vi "TMjisuan.vi"() -> ()   [LabVIEW 2018]
uses:
  <vilib>/userdefined/High Color/IMAQdx.ctl
  <vilib>/vision/driver/NI_Vision_Acquisition_Software.lvlib
  <vilib>/vision/NI_Vision_Development_Module.lvlib
panel:
  out "Frame Rate":dbl
  out "Image Number":u32
  out "位置":string
  out "appended path":path
  out "Kobs":cdb[][](array[numeric])
  in  "Stop (F)":bool caption="亮度确认"
  in  "当前增益":u32=20000 caption="Gain::Value"
  out "输出":T1(plugin-control)
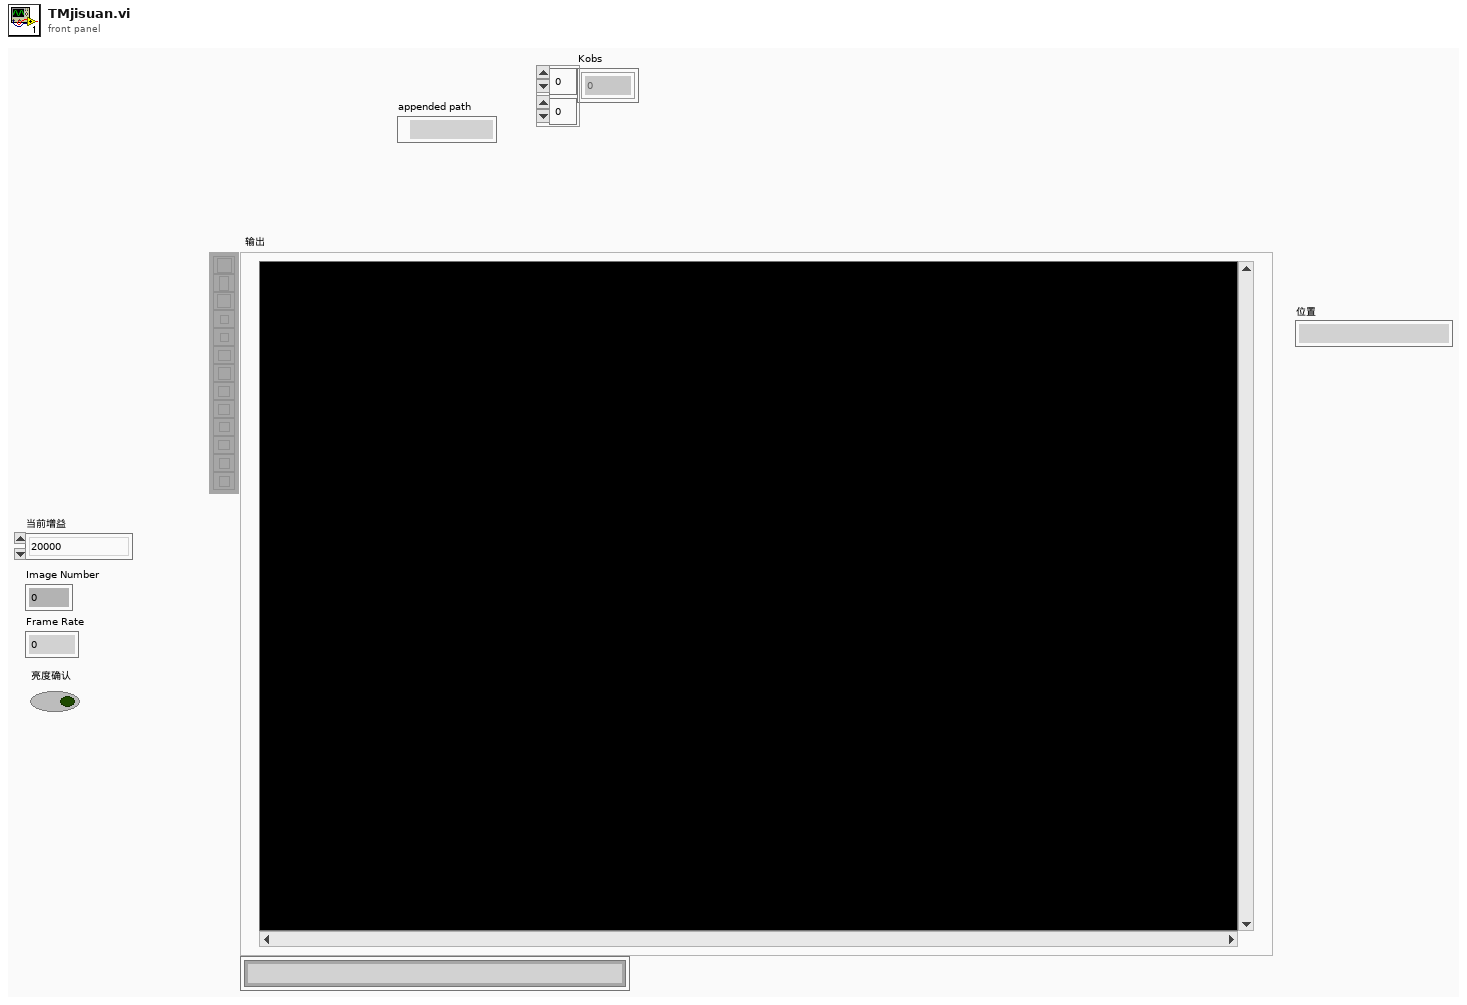
[diagram p1: front panel]
types:
  T1 = typedef "IMAQ Image.ctl" = refnum<image>
  T2 = typedef "IMAQdx.ctl" = refnum<k21>
  T3 = typedef "Image Type" = u32
  T4 = typedef "LVAllMonitorsDisplayTypeDef.ctl" = cluster{"Bounds":cluster{"Left":i16, "Top":i16, "Right":i16, "Bottom":i16}, "Depth":i16}[]
  T5 = typedef "imagedata.ctl" = cluster{"image type":i32, "image depth":i32, "image":u8[], "mask":u8[], "colors":u32[], "Rectangle":cluster{"left":i16, "top":i16, "right":i16, "bottom":i16}}
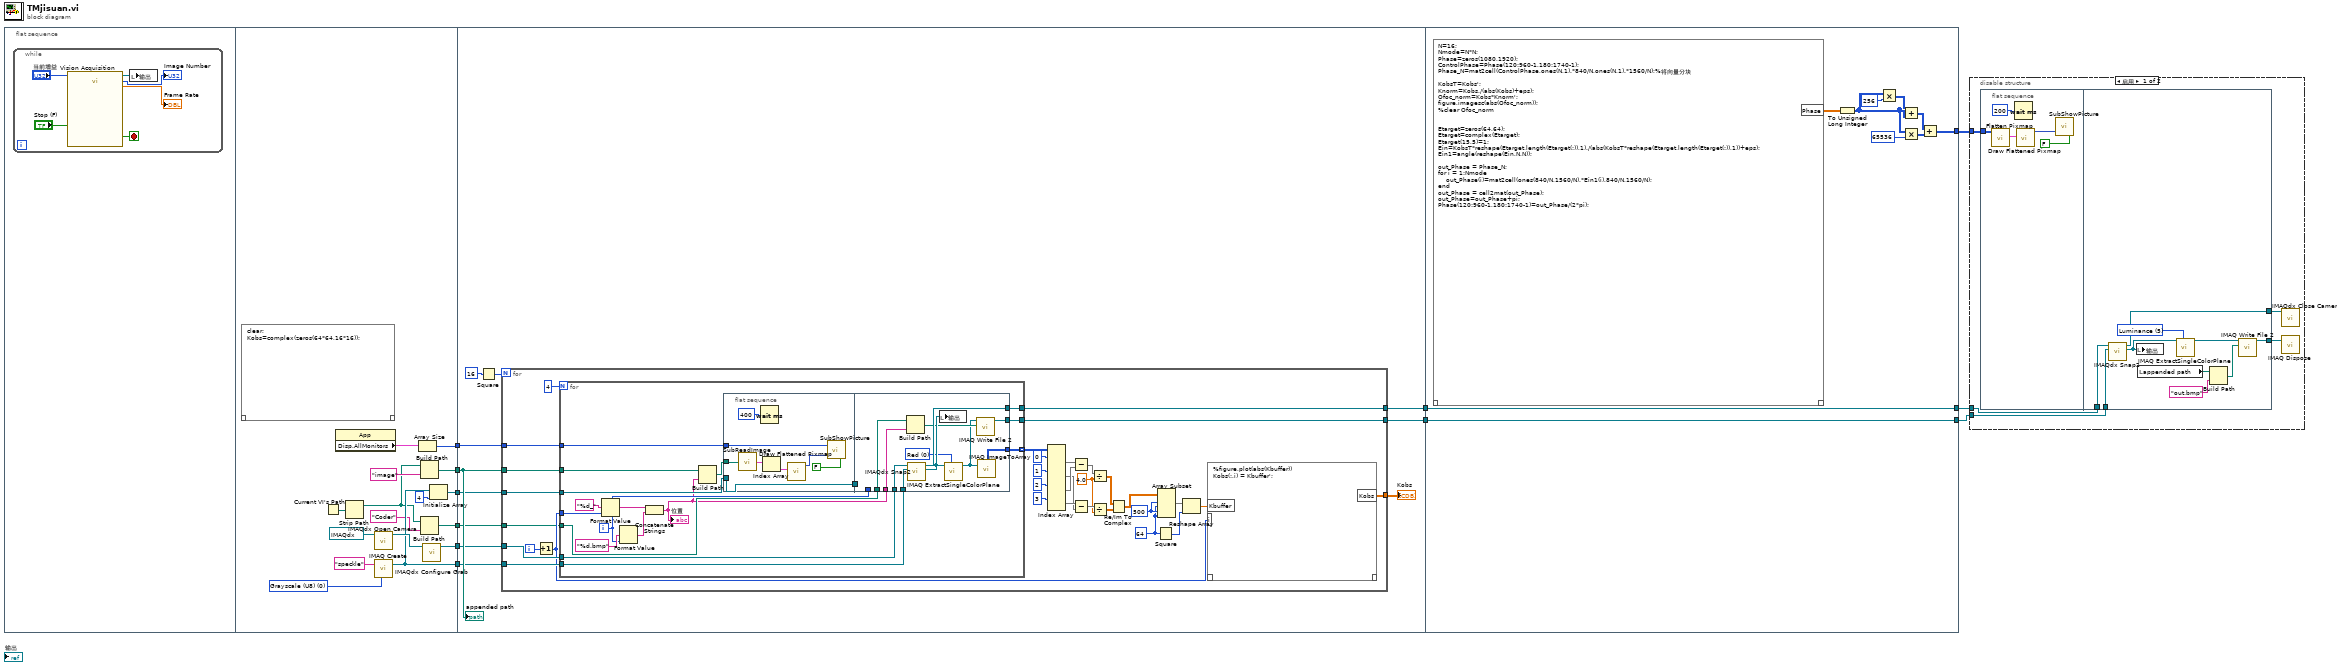
[diagram p0: block diagram]
diagram:
  n1 = flat-sequence {
    tunnel: [w30] -> w11
    tunnel: [w23] -> w10
    tunnel: [w27] -> w9
    tunnel: [w25] -> w8
    tunnel: [w21] -> w2
    tunnel: [w18] -> w1
    tunnel: w11 -> [w41]
    tunnel: w10 -> [w40]
    tunnel: w9 -> [w42]
    tunnel: w8 -> [w39]
    tunnel: [w38] -> w6
    tunnel: [w37] -> w5
    tunnel: w2 -> [w36]
    tunnel: w1 -> [w35]
    tunnel: [w122] -> w7
    tunnel: w6 -> [w121]
    tunnel: w5 -> [w120]
    tunnel: [w121] -> w4
    tunnel: [w120] -> w3
    frame #0 {
      n2 = while {
        stop <- w16 stop-if-true
        n3 = call "Vision Acquisition"("ExposureTimeAbs"="当前增益", "Stop (F)"="Stop (F)") -> ("Image Out"=w15:T1, "Image Number"=→"Image Number":u32, "Frame Rate"=→"Frame Rate":dbl, "Stopped"=w16:bool)  [unwired: 21 in, 1 out]
        n4 = local write "输出"(w15) -> ()
      }
    }
    frame #1 {
      w24 = T3 0 items=["Grayscale (U8)", "Grayscale (I16)", "Grayscale (SGL)", "Complex (CSG)", "RGB (U32)", "HSL (U32)", "RGB (U64)", "Grayscale (U16)"] ("Image Type")
      n5 = script code="clear;\nKobs=complex(zeros(64*64,16*16));"() -> ()  [unwired: 1 in, 1 out]
      n6 = Current VI's Path() -> (path=w29:path)
      n7 = property class="App"() -> ("Disp.AllMonitors"=w26:T4)  [unwired: 2 in, 2 out]
      n8 = Strip Path(path=w29) -> (stripped path=w20:path)  [unwired: 1 out]
      n9 = call <vilib>:"IMAQdx Open Camera.vi"("Session In"=T2 "cam0" ("摄像机源")) -> ("Session Out"=w32:T2)  [unwired: 9 in, 1 out]
      n10 = call "IMAQ Create"("Image Name"="speckle", "Image Type"=w24) -> ("New Image"=w23:T1)  [unwired: 3 in, 1 out]
      n11 = Array Size(array=w26) -> (size(s)=w25:i32)
      n12 = Build Path(base path=w20, name or relative path="image" ("名称或相对路径")) -> (appended path=w27:path)
      n13 = Build Path(base path=w20, name or relative path="Coder" ("名称或相对路径")) -> (appended path=w18:path)
      n14 = call <vilib>:"IMAQdx Configure Grab.vi"("Session In"=w32) -> ("Session Out"=w30:T2)  [unwired: 9 in, 1 out]
      n15 = Initialize Array(w23, 4 ("维数大小")) -> (w21:T1[])
    }
    frame #2 {
      n16 = Square(x=16) -> (x^2=w44:i32)
      n17 = for {
        N: w44 -> [_]
        tunnel: w42 -> [w74]
        tunnel: w41 -> [w73]
        tunnel: w40 -> [w72]
        tunnel: w39 -> [w71]
        tunnel: [w60] -> w38
        tunnel: [w59] -> w37
        tunnel: w36 -> [w58]
        tunnel: w35 -> [w46]
        tunnel: [w45] -> w34
        i -> [w75]
        w62 = 64 ("长度")
        w63 = 500 ("索引")
        w67 = 4.0
        n18 = Increment(x=w75) -> (x+1=w47:i32)
        n19 = for {
          N: 4 -> [_]
          tunnel: w47 -> [w94]
          tunnel: w74 -> [w89]
          tunnel: w73 -> [w86]
          tunnel: w72 -> [w85]
          tunnel: w71 -> [w87]
          tunnel: [w84] -> w60
          tunnel: [w83] -> w59
          tunnel: w58 -> [w82]
          tunnel: [w79] -> w57 mode=indexing
          tunnel: w46 -> [w78]
          i -> [w80]
          n20 = Format Value(format string="%d_" ("格式字符串"), value (0)=w94) -> (output string=w91:string)  [unwired: 1 in]
          n21 = Format Value(format string="%d.bmp" ("格式字符串"), value (0)=w80) -> (output string=w90:string)  [unwired: 1 in]
          n22 = Concatenate Strings(w91, w90) -> (w77:string)
          "位置" <- w77
          n23 = Build Path(base path=w89, name or relative path=w77) -> (appended path=w88:path)
          n24 = flat-sequence {
            tunnel: w88 -> [w97]
            tunnel: w87 -> [w96]
            tunnel: w82 -> [w95]
            tunnel: [w95] -> w81
            tunnel: w86 -> [w113]
            tunnel: w85 -> [w112]
            tunnel: [w111] -> w84
            tunnel: [w103] -> w83
            tunnel: w81 -> [_]
            tunnel: w80 -> [_]
            tunnel: [w110] -> w79
            tunnel: w78 -> [w107]
            tunnel: w77 -> [w106]
            frame #0 {
              n25 = call "SubReadImage.vi"("file or directory"=w97) -> ("Image Array"=w98:T5[])  [unwired: 3 in, 1 out]
              n26 = Wait (ms)(milliseconds to wait=400) -> ()  [unwired: 1 out]
              n27 = Index Array(array=w98) -> (element=w99:T5)  [unwired: 1 in]
              n28 = call <vilib>:"Draw Flattened Pixmap.vi"("image data"=w99) -> ("new picture"=w100:picture)  [unwired: 8 in]
              n29 = call "SubShowPicture.vi"("End"=FALSE, "Picture"=w100, "number of displays"=w96) -> ()  [unwired: 1 in]
            }
            frame #1 {
              w108 = 0 items=["Red", "Green", "Blue", "Hue", "Saturation", "Luminance", "Value", "Intensity"] ("Color Plane")
              n30 = Build Path(base path=w107, name or relative path=w106) -> (appended path=w105:path)
              n31 = call <vilib>:"IMAQdx Snap2.vi"("Image In"=w112, "Session In"=w113) -> ("Image Out"=w109:T1, "Session Out"=w111:T2)  [unwired: 7 in, 1 out]
              n32 = local write "输出"(w109) -> ()
              n33 = call "IMAQ ExtractSingleColorPlane"("Color Plane"=w108, "Image Src"=w109) -> ("Image Dst Out"=w104:T1)  [unwired: 8 in, 1 out]
              n34 = call-poly "IMAQ Write File 2"("File Path"=w105, "Image"=w104) -> ("Image Out (duplicate)"=w103:T1)  [unwired: 8 in, 1 out]
              n35 = call "IMAQ ImageToArray"("Image"=w104) -> ("Image Pixels (U8)"=w110:u8[][])  [unwired: 3 in, 4 out]
            }
          }
        }
        n36 = Index Array(array=w57, index (dim 0) #1=0 ("索引 (页)"), index (dim 0) #2=1 ("索引 (页)"), index (dim 0) #3=2 ("索引 (页)"), index (dim 0) #4=3 ("索引 (页)")) -> (element #1=w52:u8[][], element #2=w49:u8[][], element #3=w51:u8[][], element #4=w50:u8[][])  [unwired: 8 in]
        n37 = Subtract(x=w52, y=w51) -> (x-y=w69:u8[][])
        n38 = Subtract(x=w50, y=w49) -> (x-y=w68:u8[][])
        n39 = Divide(x=w69, y=w67) -> (x/y=w65:dbl[][])
        n40 = Divide(x=w68, y=w67) -> (x/y=w66:dbl[][])
        n41 = Re/Im To Complex(1:w66, 2:w65) -> (0:w64:cdb[][])
        n42 = Square(x=w62) -> (x^2=w61:i32)
        n43 = Array Subset(array=w64, index (row)=w63, length (row)=w62, index (col)=w63, length (col)=w62) -> (w70:cdb[][])
        n44 = Reshape Array(w70, w61) -> (w48:cdb[])
        n45 = script code="%figure,plot(abs(Kbuffer))\nKobs(:,i) = Kbuffer';"("Kbuffer"=w48, "i"=w47) -> ("Kobs"=w45:cdb[][])  [unwired: 1 in, 1 out]
      }
      "Kobs" <- w34
      "appended path" <- w42
    }
    frame #3 {
      n46 = script code="N=16;\nNmode=N*N;\nPhase=zeros(1080,1920);\nControlPhase=Phase(120:960-1,180:1740-1);\nPhase_N=mat2cell(ControlPhase,ones(N,1).*840/N,ones(N,1).*1560/N);%将向量分块\n\nKobsT=Kobs';\nKnorm=Kobs./(abs(Kobs)+eps);\nOfoc_norm=Kobs*Knorm';\nfigure,imagesc(abs(Ofoc_norm));\n%clear Ofoc_norm\n\n\nEtarget=zeros(64,64);\nEtarget=complex(Etarget);\nEtarget(15,5)=1;\nEin=KobsT*reshape(Etarget,length(Etarget(:)),1)./(abs(KobsT*reshape(Etarget,length(Etarget(:)),1))+eps);\nEin1=angle(reshape(Ein,N,N));\n\nout_Phase = Phase_N;\nfor i = 1:Nmode\n    out_Phase(i)=mat2cell(ones(840/N,1560/N).*Ein1(i),840/N,1560/N);\nend\nout_Phase = cell2mat(out_Phase);\nout_Phase=out_Phase+pi;\nPhase(120:960-1,180:1740-1)=out_Phase/(2*pi);"() -> ("Phase"=w123:dbl[][])  [unwired: 1 in, 1 out]
      n47 = To Unsigned Long Integer(number=w123) -> (unsigned 32bit integer=w118:u32[][])
      n48 = Multiply(x=w118, y=256) -> (x*y=w116:u32[][])
      n49 = Add(x=w118, y=w116) -> (x+y=w115:u32[][])
      n50 = Multiply(x=w118, y=65536) -> (x*y=w114:u32[][])
      n51 = Add(x=w115, y=w114) -> (x+y=w122:u32[][])
    }
  }
  n52 = disable-structure shown="启用" {
    disable-tunnel: w7 -> [w128 _]
    disable-tunnel: w4 -> [w127 _]
    disable-tunnel: w3 -> [w126 _]
    frame Enabled {
      n53 = flat-sequence {
        tunnel: w128 -> [w130]
        tunnel: w127 -> [w143]
        tunnel: w126 -> [w142]
        tunnel: [w141] -> w125
        tunnel: [w137] -> w124
        frame #0 {
          n54 = call <vilib>:"Flatten Pixmap.vi"("24-bit pixmap"=w130) -> ("image data"=w131:T5)  [unwired: 10 in]
          n55 = Wait (ms)(milliseconds to wait=200) -> ()  [unwired: 1 out]
          n56 = call <vilib>:"Draw Flattened Pixmap.vi"("image data"=w131) -> ("new picture"=w132:picture)  [unwired: 8 in]
          n57 = call "SubShowPicture.vi"("End"=FALSE, "Picture"=w132) -> ()  [unwired: 2 in]
        }
        frame #1 {
          w139 = 5 items=["Red", "Green", "Blue", "Hue", "Saturation", "Luminance", "Value", "Intensity"] ("Color Plane")
          n58 = call <vilib>:"IMAQdx Snap2.vi"("Image In"=w142, "Session In"=w143) -> ("Image Out"=w140:T1, "Session Out"=w141:T2)  [unwired: 7 in, 1 out]
          n59 = local write "输出"(w140) -> ()
          n60 = local read "appended path"() -> (w135:path)
          n61 = call "IMAQ ExtractSingleColorPlane"("Color Plane"=w139, "Image Src"=w140) -> ("Image Dst Out"=w138:T1)  [unwired: 8 in, 1 out]
          n62 = Build Path(base path=w135, name or relative path="out.bmp" ("名称或相对路径")) -> (appended path=w136:path)
          n63 = call-poly "IMAQ Write File 2"("File Path"=w136, "Image"=w138) -> ("Image Out (duplicate)"=w137:T1)  [unwired: 8 in, 1 out]
        }
      }
      n64 = call <vilib>:"IMAQdx Close Camera.vi"("Session In"=w125) -> ()  [unwired: 10 in, 1 out]
      n65 = call "IMAQ Dispose"("Image"=w124) -> ()  [unwired: 5 in, 1 out]
    }
    frame Disabled {
    }
  }
